vi "Get Actual Power.vi"(8 "error in":errorcluster, 10 "MCU Selector":T1, 11 "HSU MCU V2 Monitor CFG in":refnum<class "HSU MCU V2 Monitor CFG.lvclass">) -> (0 "error out":errorcluster, 1 "Torque":dbl format="%#_g Nm", 2 "Power":dbl format="%#_g W", 3 "HSU MCU V2 Monitor CFG out":refnum<class "HSU MCU V2 Monitor CFG.lvclass">)   [LabVIEW 2023, in "HSU MCU V2 Monitor CFG.lvclass"]
uses:
  HSU MCU V2 Monitor CFG.lvclass
  MCU Selector.ctl
  HSU MCU V2 Monitor CFG.lvclass/HSU MCU V2 Monitor CFG.ctl
  Protocols/ICAN/ICAN.lvclass
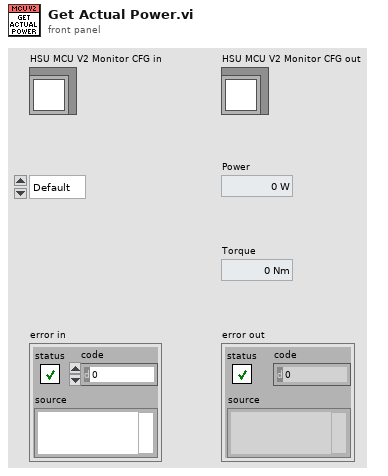
[diagram p1: front panel]
types:
  T1 = typedef "MCU Selector.ctl" = enum16{"Default", "MCU1", "MCU2", "MCU3", "MCU4", "MCU5", "MCU6", "MCU7", "MCU8"}
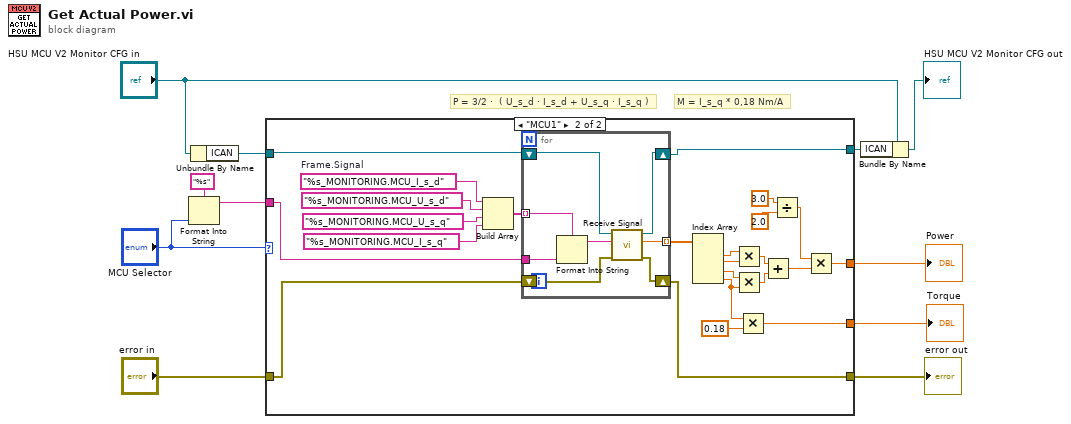
[diagram p0: block diagram]
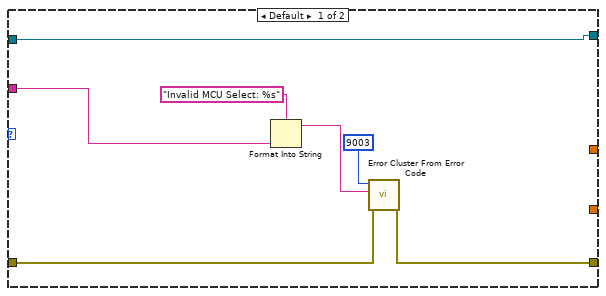
[diagram p2: hidden frame]
diagram:
  # "M = I_s_q * 0,18 Nm/A"
  # "P = 3/2 ·  ( U_s_d · I_s_d + U_s_q · I_s_q )"
  n1 = Format Into String(format string="%s", "MCU Selector") -> (resulting string=w8:string)  [unwired: 2 in, 1 out]
  n2 = Unbundle By Name("HSU MCU V2 Monitor CFG in") -> ("ICAN"=w7:refnum<class "ICAN.lvclass">)
  n3 = case shown="\"MCU1\"" "MCU Selector" {
    tunnel: "error in" -> [w18 w35]
    tunnel: [w17 w23] -> w5
    tunnel: w8 -> [w13 w37]
    tunnel: w7 -> [w12 w36]
    tunnel: [_ w24] -> w6
    tunnel: [w12 w22] -> w4
    tunnel: [_ w19] -> w1
    frame Default {
      n4 = Format Into String(format string="Invalid MCU Select: %s" ("error message (\"\")"), w13) -> (resulting string=w15:string)  [unwired: 2 in, 1 out]
      n5 = call <vilib>:"Error Cluster From Error Code.vi"("error in (no error)"=w18, "error message (\"\")"=w15, "error code (0)"=9003) -> ("error out"=w17:errorcluster)  [unwired: 6 in]
    }
    frame "MCU1" {
      w42 = "%s_MONITORING.MCU_I_s_d"  # Frame.Signal
      n6 = Build Array(w42, "%s_MONITORING.MCU_U_s_d" ("Frame.Signal"), "%s_MONITORING.MCU_U_s_q" ("Frame.Signal"), "%s_MONITORING.MCU_I_s_q" ("Frame.Signal")) -> (w38:string[])
      n7 = for {
        tunnel: w38 -> [w49] mode=indexing
        tunnel: w37 -> [w50]
        tunnel: [w44] -> w34 mode=indexing
        shift-right: [w45] -> w23
        shift-left: w35 -> [w46]
        shift-right: [w43] -> w22
        shift-left: w36 -> [w48]
        n8 = Format Into String(format string=w49, w50) -> (resulting string=w47:string)  [unwired: 2 in, 1 out]
        n9 = call-dynamic "Receive Signal.vi"("error in"=w46, "Frame.Signal"=w47, "ICommunicate in"=w48) -> ("error out"=w45:errorcluster, "Value"=w44:dbl, "ICommunicate out"=w43:refnum<class "ICAN.lvclass">)  [unwired: 6 in]
      }
      n10 = Index Array(array=w34) -> (element #1=w33:dbl, element #2=w32:dbl, element #3=w31:dbl, element #4=w21:dbl)  [unwired: 4 in]
      n11 = Multiply(x=w33, y=w32) -> (x*y=w30:dbl)
      n12 = Multiply(x=w31, y=w21) -> (x*y=w29:dbl)
      n13 = Multiply(x=w21, y=0.18) -> (x*y=w19:dbl)
      n14 = Add(x=w30, y=w29) -> (x+y=w28:dbl)
      n15 = Divide(x=3.0, y=2.0) -> (x/y=w25:dbl)
      n16 = Multiply(x=w25, y=w28) -> (x*y=w24:dbl)
    }
  }
  "error out" <- w5
  "Power" <- w6
  "Torque" <- w1
  n17 = Bundle By Name(cluster="HSU MCU V2 Monitor CFG in", "ICAN"=w4) -> (→"HSU MCU V2 Monitor CFG out":refnum<class "HSU MCU V2 Monitor CFG.lvclass">)
